vi "Unflatten Report Parameters.vi"(11 "Parameter String":string) -> (1 "Defaults loaded":bool, 2 "Error":bool, 3 "Report Parameters":T1={"REPORT_TDR_PATH"="", "ROOT_PATH"="", "PLOT1_TDM_PATH"="", "REPORT_PDF_PATH"="", "PLOT1_RUN_ID"=1, "PLOT_STYLE"=0, "COMPANY_ID_TXT"="", "DATETIME_TXT"="", "OPERATOR_TXT"="", "SERIALNUMBER_TXT"="", "MODELNUMBER_TXT"="", "SEQID_TXT"="", "INSTRID_TXT"="", "CUSTOMTXT 1"="", "CUSTOMTXT 2"="", "CUSTOMTXT 3"="", "CUSTOMTXT 4"="", "CUSTOMTXT 5"="", "CUSTOMTXT 6"="", "CUSTOMTXT 7"="", "CUSTOMTXT 8"="", "CUSTOMTXT 9"="", "CUSTOMTXT 10"="", "PLOT1_LABEL_TXT"="", "PLOT1_Y_TXT"="", "PLOT1_X_TXT"="", "PLOT2_LABEL_TXT"="", "PLOT2_Y_TXT"="", "PLOT2_X_TXT"="", "REPORTFOOTER"="", "PLOT1_FORMAT"=0, "PLOT1_LINETYPE"=1, "PLOT1_CURVES"=[], "PLOT1_AUTO_X"=1, "PLOT1_XMIN"=0.0, "PLOT1_XMAX"=0.0, "PLOT1_X_UNIT"=2, "PLOT1_AUTO_Y"=1, "PLOT1_YMIN"=0.0, "PLOT1_YMAX"=0.0, "PLOT2_FORMAT"=0, "PLOT2_LINETYPE"=1, "PLOT2_CURVES"=[], "PLOT2_AUTO_X"=1, "PLOT2_XMIN"=0.0, "PLOT2_XMAX"=0.0, "PLOT2_X_UNIT"=2, "PLOT2_AUTO_Y"=1, "PLOT2_YMIN"=0.0, "PLOT2_YMAX"=0.0, "PRINTER"="", "CUSTOMTXT 11"="", "CUSTOMTXT 12"="", "CUSTOMTXT 13"="", "CUSTOMTXT 14"="", "CUSTOMTXT 15"="", "CUSTOMTXT 16"="", "CUSTOMTXT 17"="", "CUSTOMTXT 18"="", "CUSTOMTXT 19"="", "CUSTOMTXT 20"="", "Custom_Count"=1, "PLOT1_MARKERS"=[], "PLOT2_MARKERS"=[], "S2P"=1, "ASCII"=1} {"PLOT2_X_UNIT" items=["Hz", "kHz", "MHz", "GHz"]; "PLOT2_FORMAT" items=["Log Magnitude", "Phase", "Delay", "Linear Magnitude", "VSWR", "Insertion Loss", "Isolation", "Return Loss", "Expanded Phase"]; "PLOT1_X_UNIT" items=["Hz", "kHz", "MHz", "GHz"]; "PLOT1_FORMAT" items=["Log Magnitude", "Phase", "Delay", "Linear Magnitude", "VSWR", "Insertion Loss", "Isolation", "Return Loss", "Expanded Phase"]; "PLOT_STYLE" items=["PDF", "HTML"]}, 5 "Test Version":string)   [LabVIEW 2011]
uses:
  server/DIAdem/Datasheet/Datasheet Sxx Parameters.ctl
  server/DIAdem/Datasheet/Datasheet Sxx Plot Formats.ctl
  server/DIAdem/Datasheet/Datasheet Sxx Plot Control.ctl
  server/DIAdem/Datasheet/Datasheet Sxx Frequency Units.ctl
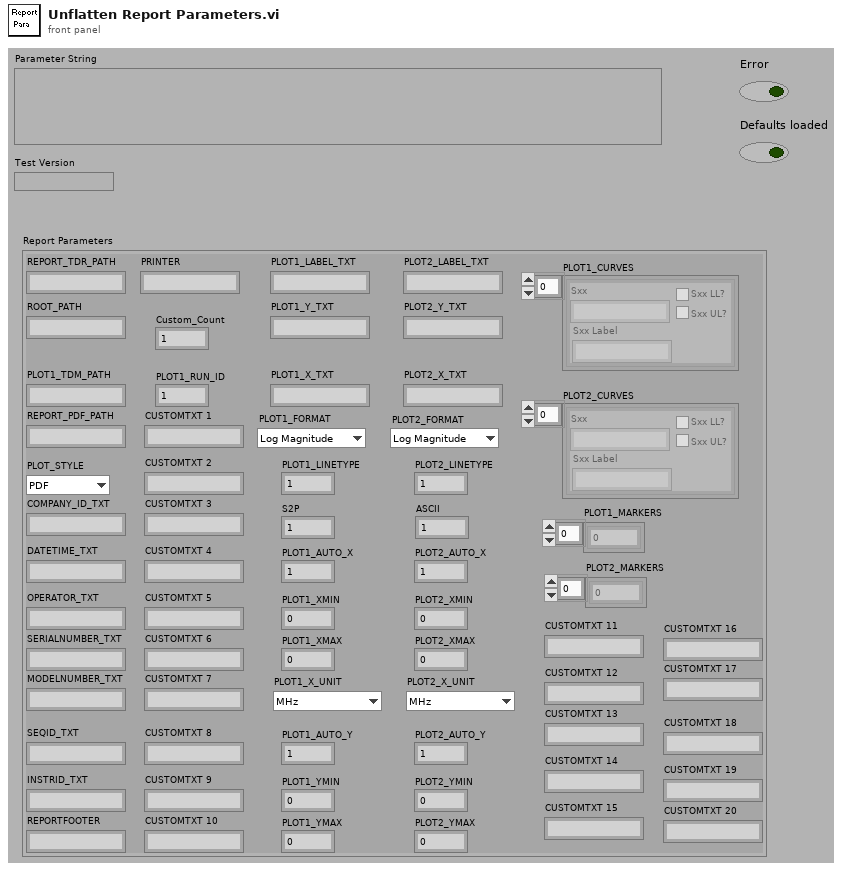
[diagram p1: front panel]
types:
  T1 = typedef "DATASHEET Sxx Parameters.ctl" = cluster{"REPORT_TDR_PATH":string, "ROOT_PATH":string, "PLOT1_TDM_PATH":string, "REPORT_PDF_PATH":string, "PLOT1_RUN_ID":i32, "PLOT_STYLE":u16, "COMPANY_ID_TXT":string, "DATETIME_TXT":string, "OPERATOR_TXT":string, "SERIALNUMBER_TXT":string, "MODELNUMBER_TXT":string, "SEQID_TXT":string, "INSTRID_TXT":string, "CUSTOMTXT 1":string, "CUSTOMTXT 2":string, "CUSTOMTXT 3":string, "CUSTOMTXT 4":string, "CUSTOMTXT 5":string, "CUSTOMTXT 6":string, "CUSTOMTXT 7":string, "CUSTOMTXT 8":string, "CUSTOMTXT 9":string, "CUSTOMTXT 10":string, "PLOT1_LABEL_TXT":string, "PLOT1_Y_TXT":string, "PLOT1_X_TXT":string, "PLOT2_LABEL_TXT":string, "PLOT2_Y_TXT":string, "PLOT2_X_TXT":string, "REPORTFOOTER":string, "PLOT1_FORMAT":T2, "PLOT1_LINETYPE":i32, "PLOT1_CURVES":T3[], "PLOT1_AUTO_X":i32, "PLOT1_XMIN":dbl, "PLOT1_XMAX":dbl, "PLOT1_X_UNIT":T4, "PLOT1_AUTO_Y":i32, "PLOT1_YMIN":dbl, "PLOT1_YMAX":dbl, "PLOT2_FORMAT":T2, "PLOT2_LINETYPE":i32, "PLOT2_CURVES":T3[], "PLOT2_AUTO_X":i32, "PLOT2_XMIN":dbl, "PLOT2_XMAX":dbl, "PLOT2_X_UNIT":T4, "PLOT2_AUTO_Y":i32, "PLOT2_YMIN":dbl, "PLOT2_YMAX":dbl, "PRINTER":string, "CUSTOMTXT 11":string, "CUSTOMTXT 12":string, "CUSTOMTXT 13":string, "CUSTOMTXT 14":string, "CUSTOMTXT 15":string, "CUSTOMTXT 16":string, "CUSTOMTXT 17":string, "CUSTOMTXT 18":string, "CUSTOMTXT 19":string, "CUSTOMTXT 20":string, "Custom_Count":i32, "PLOT1_MARKERS":dbl[], "PLOT2_MARKERS":dbl[], "S2P":i32, "ASCII":i32}
  T2 = typedef "DATASHEET Sxx Plot Formats.ctl" = u16
  T3 = typedef "DATASHEET Sxx Plot Control.ctl" = cluster{"Sxx":string, "Sxx LL?":bool, "Sxx UL?":bool, "Sxx Label":string}
  T4 = typedef "DATASHEET Sxx Frequency Units.ctl" = u16
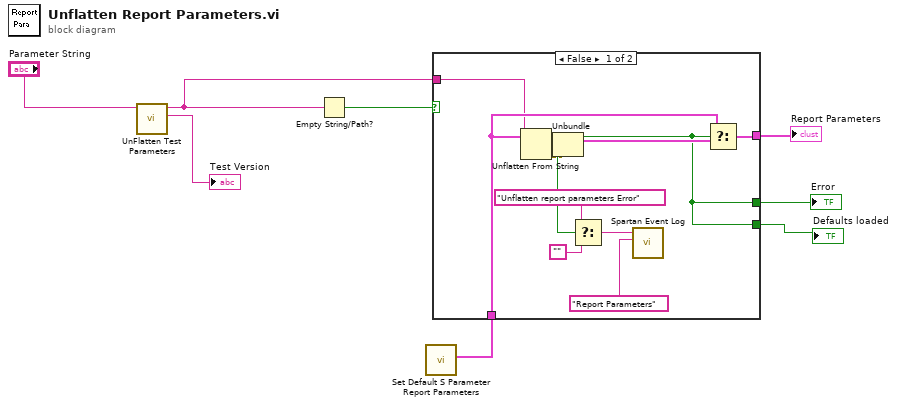
[diagram p0: block diagram]
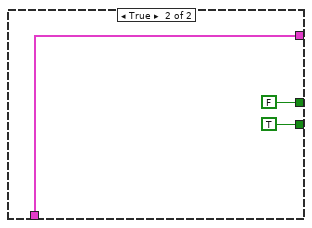
[diagram p2: hidden frame]
diagram:
  n1 = call "UnFlatten Test Parameters.vi"("Flattened Test Parameters with Version (\"\")"="Parameter String") -> ("Test Version"=→"Test Version":string, "Flat Test Parameters"=w3:string)  [unwired: 1 in, 4 out]
  n2 = Empty String/Path?(string/path=w3) -> (empty?=w4:bool)
  n3 = call "Set Default S Parameter Report Parameters.vi"() -> ("Report Variables"=w5:T1)  [unwired: 11 out]
  n4 = case shown="False" w4 {
    tunnel: w5 -> [w17 w21]
    tunnel: [w16 w21] -> w8
    tunnel: [w13 FALSE ("err")] -> w7
    tunnel: [w13 TRUE ("err")] -> w6
    tunnel: w3 -> [w15 _]
    frame False {
      n5 = Unflatten From String(type=w17, binary string=w15) -> (value=w18:T1, error out=w9:errorcluster)  [unwired: 1 in, 3 out]
      n6 = Unbundle(w9) -> ("status"=w13:bool)  [unwired: 2 out]
      n7 = Select(t="Unflatten report parameters Error" ("name (unnamed)"), s=w13, f="") -> (s? t:f=w12:string)
      n8 = call "Spartan Event Log.vi"("module (\"\")"="Report Parameters" ("name (unnamed)"), "message (\"\")"=w12) -> ()  [unwired: 3 in, 4 out]
      n9 = Select(t=w17, s=w13, f=w18) -> (s? t:f=w16:T1)
    }
    frame True {
    }
  }
  "Report Parameters" <- w8
  "Error" <- w7
  "Defaults loaded" <- w6
